vi "_Launch Dynamic VI.vi"(0 "VI Name":path) -> (1 "VI Refnum":refnum<vi>)   [LabVIEW 2015]
panel:
  out "path":path
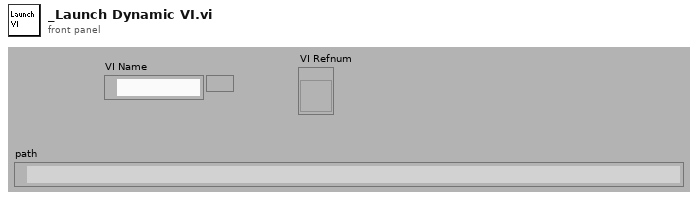
[diagram p1: front panel]
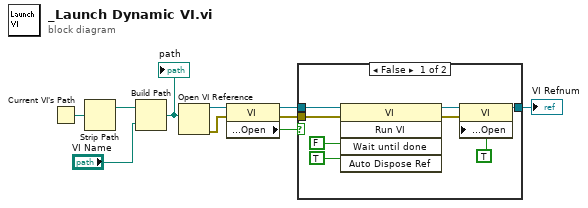
[diagram p0: block diagram]
diagram:
  n1 = Current VI's Path() -> (path=w9:path)
  n2 = Strip Path(path=w9) -> (stripped path=w10:path)  [unwired: 1 out]
  n3 = Build Path(base path=w10, name or relative path="VI Name") -> (appended path=w8:path)
  "path" <- w8
  n4 = Open VI Reference(vi path=w8) -> (vi reference=w6:refnum<vi>, error out=w3:errorcluster)  [unwired: 1 in, 4 out]
  n5 = property class="VI"(reference=w6, error in=w3) -> (reference out=w5:refnum<vi>, error out=w4:errorcluster, "Front Panel.Open"=w2:bool)
  n6 = case shown="False" w2 {
    tunnel: w5 -> [w13 w19]
    tunnel: w4 -> [w12 _]
    tunnel: [w11 w19] -> w1
    frame False {
      n7 = invoke class="VI" method="Run VI"(reference=w13, error in=w12, "Wait until done"=FALSE, "Auto Dispose Ref"=TRUE ("Auto Dispose Reference")) -> (reference out=w16:refnum<vi>, error out=w17:errorcluster)  [unwired: 1 in, 3 out]
      n8 = property class="VI"(reference=w16, error in=w17, "Front Panel.Open"=TRUE ("Front Panel Window:Open")) -> (reference out=w11:refnum<vi>)  [unwired: 1 out]
    }
    frame True {
    }
  }
  "VI Refnum" <- w1
